vi "Pratik3-Case1.vi"() -> ()   [LabVIEW 2024]
panel:
  out "Frequency(mHz)":dbl
  out "number":u32
  out "Enum":T1(ring)=enum."Operational Mode"
  out "Message":string
  out "subarray(EPS mode)":bool[](array[boolean])
  out "Period Value Phase 1 (ms)":dbl
  out "Current Value Phase1":dbl
  out "Voltage Value Phase1":dbl
  in  "Input String":string
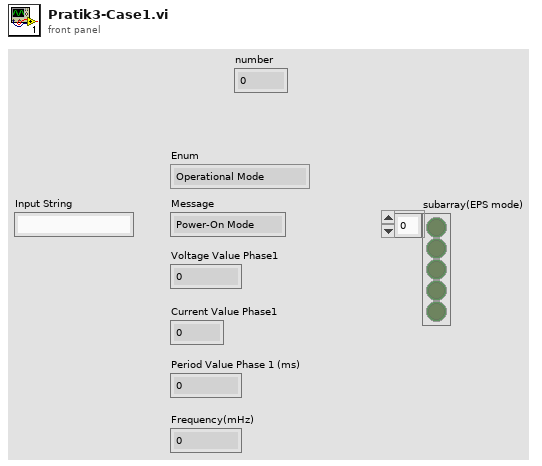
[diagram p1: front panel]
types:
  T1 = enum8{"Power-On Mode", "Maintenance Mode", "Operational Mode", "Emergency Mode"}
  T2 = enum16{"Power-On Mode", "Maintenance Mode", "Operational Mode", "Emergency Mode"}
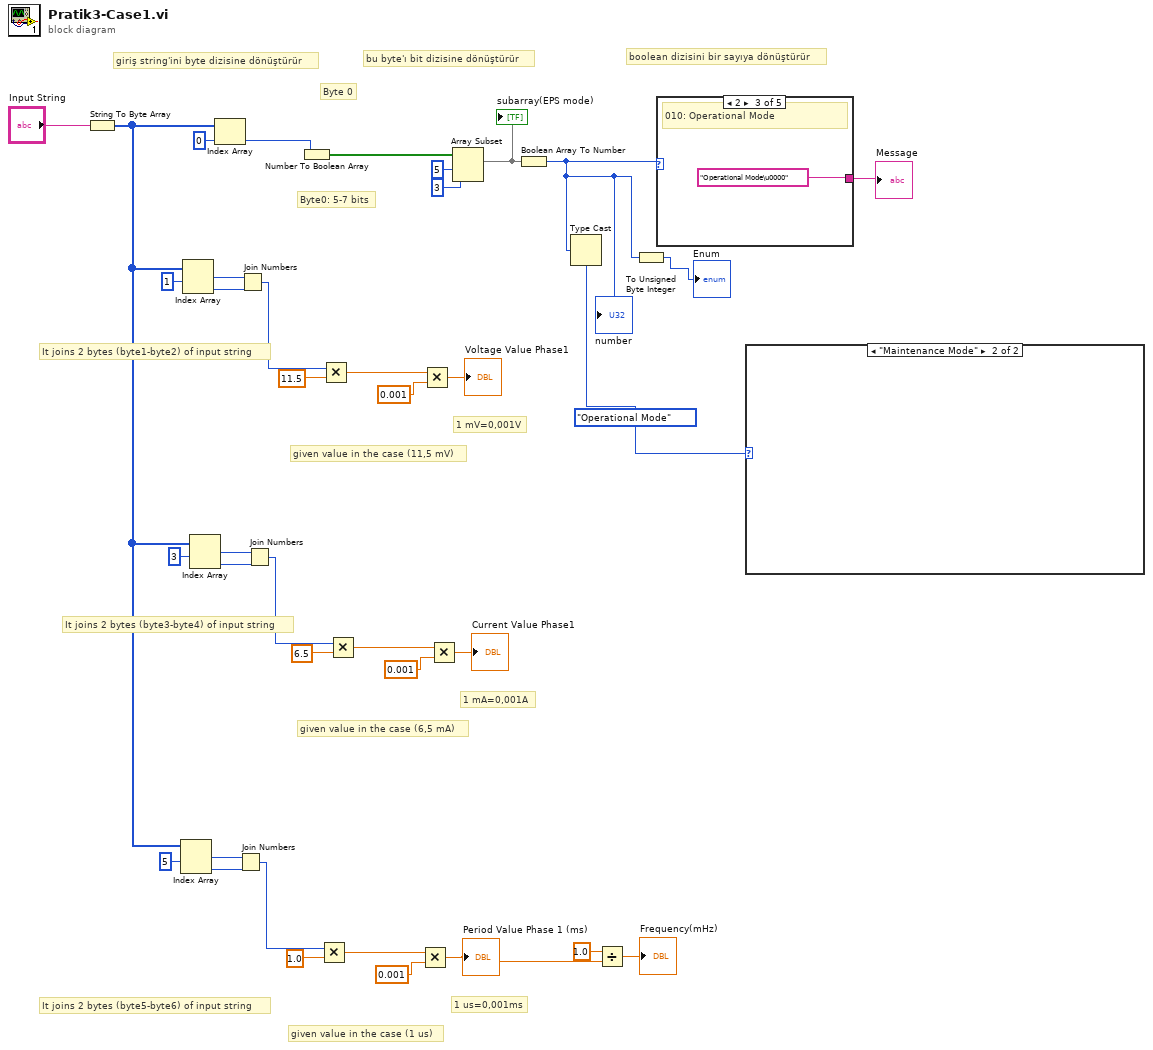
[diagram p0: block diagram]
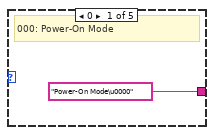
[diagram p3: hidden frame]
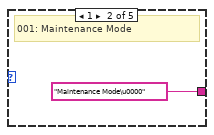
[diagram p4: hidden frame]
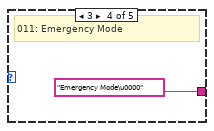
[diagram p5: hidden frame]
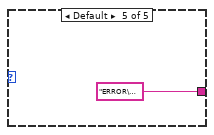
[diagram p6: hidden frame]
diagram:
  w6 = T2."Operational Mode"
  # "boolean dizisini bir sayıya dönüştürür"
  # "Byte0: 5-7 bits"
  # "bu byte'ı bit dizisine dönüştürür"
  # "Byte 0"
  # "giriş string'ini byte dizisine dönüştürür"
  # "given value in the case (1 us)"
  # "It joins 2 bytes (byte5-byte6) of input string"
  # "1 us=0,001ms"
  # "given value in the case (6,5 mA)"
  # "It joins 2 bytes (byte3-byte4) of input string"
  # "1 mA=0,001A"
  # "given value in the case (11,5 mV)"
  # "It joins 2 bytes (byte1-byte2) of input string"
  # "1 mV=0,001V"
  n1 = String To Byte Array(string="Input String") -> (unsigned byte array=w9:u8[])
  n2 = Index Array "Index Array"(array=w9, index #1=5 ("index")) -> (element #1=w20:u8, element #2=w19:u8)  [unwired: 1 in]
  n3 = Index Array "Index Array"(array=w9, index #1=1 ("index")) -> (element #1=w36:u8, element #2=w35:u8)  [unwired: 1 in]
  n4 = Index Array "Index Array"(array=w9, index #1=3 ("index")) -> (element #1=w28:u8, element #2=w27:u8)  [unwired: 1 in]
  n5 = Index Array "Index Array"(array=w9, index=0) -> (element=w13:u8)
  n6 = Join Numbers(hi=w20, lo=w19) -> ((hi.lo)=w15:u16)
  n7 = Join Numbers(hi=w36, lo=w35) -> ((hi.lo)=w31:u16)
  n8 = Join Numbers(hi=w28, lo=w27) -> ((hi.lo)=w23:u16)
  n9 = Number To Boolean Array(number=w13) -> (Boolean array=w12:bool[])
  n10 = Multiply(x=w15, y=1.0) -> (x*y=w17:dbl)
  n11 = Multiply(x=w31, y=11.5) -> (x*y=w33:dbl)
  n12 = Multiply(x=w23, y=6.5) -> (x*y=w25:dbl)
  n13 = Multiply(x=w17, y=0.001) -> (x*y=w1:dbl)
  "Period Value Phase 1 (ms)" <- w1
  n14 = Multiply(x=w33, y=0.001) -> (x*y=→"Voltage Value Phase1":dbl)
  n15 = Multiply(x=w25, y=0.001) -> (x*y=→"Current Value Phase1":dbl)
  n16 = Array Subset "Array Subset"(array=w12, index=5, length=3) -> (w8:bool[])
  "subarray(EPS mode)" <- w8
  n17 = Boolean Array To Number(Boolean array=w8) -> (number=w5:u32)
  "number" <- w5
  n18 = Type Cast(type=w6, x=w5) -> ()  [unwired: 1 out]
  n19 = Divide(x=1.0, y=w1) -> (x/y=→"Frequency(mHz)":dbl)
  n20 = To Unsigned Byte Integer(number=w5) -> (unsigned 8bit integer=→"Enum":u8)
  n21 = case shown="2" w5 {
    tunnel: ["Power-On Mode\u0000" "Maintenance Mode\u0000" "Operational Mode\u0000" "Emergency Mode\u0000" "ERROR\u0000"] -> w7
    frame 0 {
      # "000: Power-On Mode"
    }
    frame 1 {
      # "001: Maintenance Mode"
    }
    frame 2 {
      # "010: Operational Mode"
    }
    frame 3 {
      # "011: Emergency Mode"
    }
    frame Default {
    }
  }
  "Message" <- w7
  n22 = case shown="\"Maintenance Mode\"" w6 {
    frame "Power-On Mode", Default {
    }
    frame "Maintenance Mode" {
    }
  }
